vi "CmdExe.Callback for .NET OutputDataRecieved Event.vi"(4 "StdOut":refnum<vi>, 5 "Event Data":cluster{"sender":refnum<k24>, "e":refnum<k24>}, 6 "Control Ref":refnum<k24>, 7 "Event Common Data":T1) -> ()   [LabVIEW 2018]
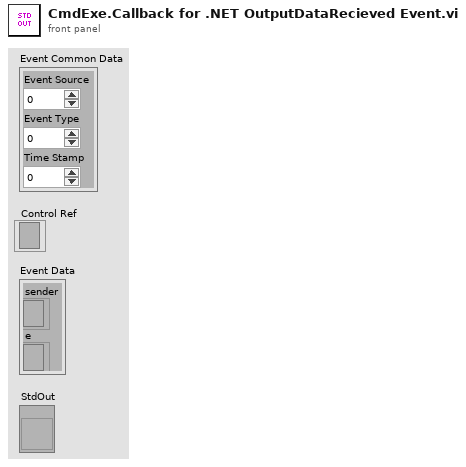
[diagram p1: front panel]
types:
  T1 = cluster{"Event Source":i32, "Event Type":u32, "Time Stamp":u32}
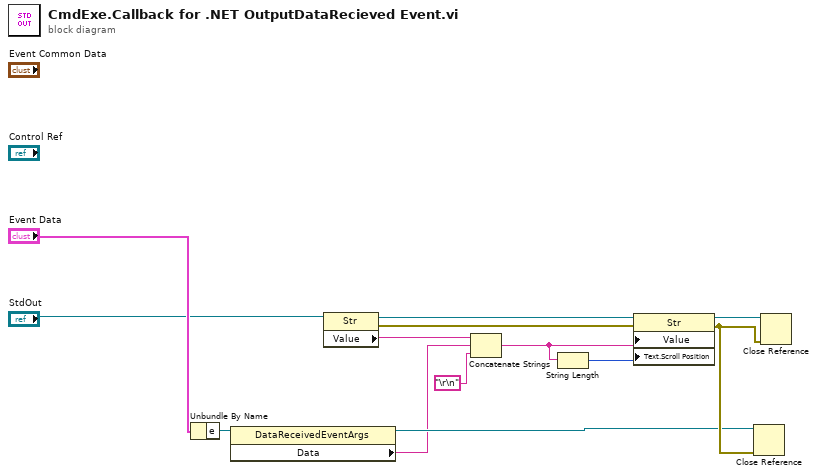
[diagram p0: block diagram]
diagram:
  n1 = Unbundle By Name("Event Data") -> ("e"=w12:refnum<k24>)
  n2 = property class="DataReceivedEventArgs"(reference=w12) -> (reference out=w9:refnum<k24>, "Data"=w6:string)  [unwired: 1 in, 1 out]
  n3 = property class="Str"(reference="StdOut") -> (reference out=w5:refnum<vi>, error out=w4:errorcluster, "Value"=w7:string)  [unwired: 1 in]
  n4 = Concatenate Strings(w7, w6, "\r\n") -> (w2:string)
  n5 = String Length(string=w2) -> (length=w1:i32)
  n6 = property class="Str"(reference=w5, error in=w4, "Value"=w2, "Text.Scroll Position"=w1) -> (reference out=w11:refnum<vi>, error out=w10:errorcluster)
  n7 = Close Reference(reference=w9, error in (no error)=w10) -> ()  [unwired: 1 out]
  n8 = Close Reference(reference=w11, error in (no error)=w10) -> ()  [unwired: 1 out]
